vi "Pre Launch Init.vi"(11 "Main Display in":refnum<class "Main Display.lvclass">) -> (0 "error out":errorcluster, 3 "Main Display out":refnum<class "Main Display.lvclass">)   [LabVIEW 2016, in "Assert API Components.lvlib" / "Assert Display.lvlib" / "Main Display.lvlib" / "Main Display.lvclass"]
doc: "(<B>Filename</B>: Actor Framework.lvlib:Actor.lvclass:Pre Launch Init.vi)\n\nDefines behavior that occurs after the Launch Nested Actor method is invoked but before the actor's Actor Core method begins running.\n\nBy default, this method does nothing. A descendant class may override it to define behavior."
uses:
  Main Display.lvclass
  Main Display.lvclass/Main Display.ctl
  Display Configurations/Standard Display Configuration/Standard Display Configuration.lvclass
  D:/Work/Projects/actor_assert_api/Core/Main Display/Display Configurations/Base Display Configuration.lvclass
  Base UI Component/Base UI Component/Base UI Component.lvclass
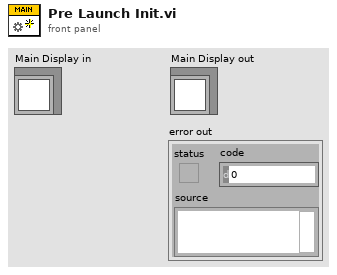
[diagram p1: front panel]
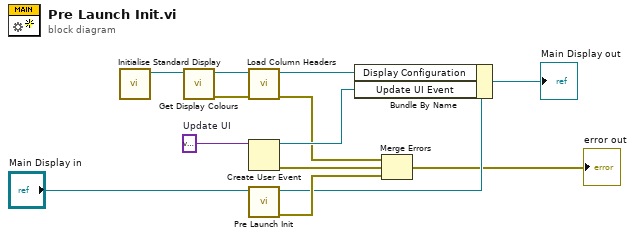
[diagram p0: block diagram]
diagram:
  w10 = variant  # Update UI
  n1 = call "Initialise Standard Display.vi"() -> ("Standard Display Configuration out"=w3:refnum<class "Standard Display Configuration.lvclass">)  [unwired: 11 in]
  n2 = call-dynamic "Get Display Colours.vi"("Standard Display Configuration in"=w3) -> ("error out"=w1:errorcluster, "Standard Display Configuration out"=w2:refnum<class "Standard Display Configuration.lvclass">)  [unwired: 9 in]
  n3 = call-dynamic "Load Column Headers.vi"("error in (no error)"=w1, "Standard Display Configuration in"=w2) -> ("error out"=w4:errorcluster, "Standard Display Configuration out"=w5:refnum<class "Standard Display Configuration.lvclass">)  [unwired: 8 in]
  n4 = Create User Event(user event datatype=w10) -> (user event=w8:refnum<user-event>, error out=w6:errorcluster)  [unwired: 1 in]
  n5 = call-parent "Pre Launch Init.vi"("Base UI Component in"="Main Display in") -> ("error out"=w13:errorcluster, "Base UI Component out"=w12:refnum<class "Main Display.lvclass">)  [unwired: 9 in]
  n6 = Bundle By Name(cluster=w12, "Display Configuration"=w5, "Update UI Event"=w8) -> (→"Main Display out":refnum<class "Main Display.lvclass">)
  n7 = Merge Errors(w4, w6, w13) -> (→"error out":errorcluster)
